vi "Simple Polar Plot.vi"() -> ()   [LabVIEW 2017]
doc: "Uses the Polar Plot with Point Options VI to draw a polar plot in a picture indicator."
panel:
  in  "Plot Color":u32(colorbox)=16715776
  in  "Grid Color":u32(colorbox)
  in  "Visible Section":u16(ring)=8
  in  "Stop":bool
  out "2D Picture":picture
  # "Overview: Demonstrates how to display and customize a polar plot using the Polar Plot with Point Options VI.\nInstructions:\n1. Run the VI.\n2. Change the Cosmetic Options to modify the visible area and appearance of the plot.\n3. Click Stop to stop the VI."
  # "Cosmetic Options"
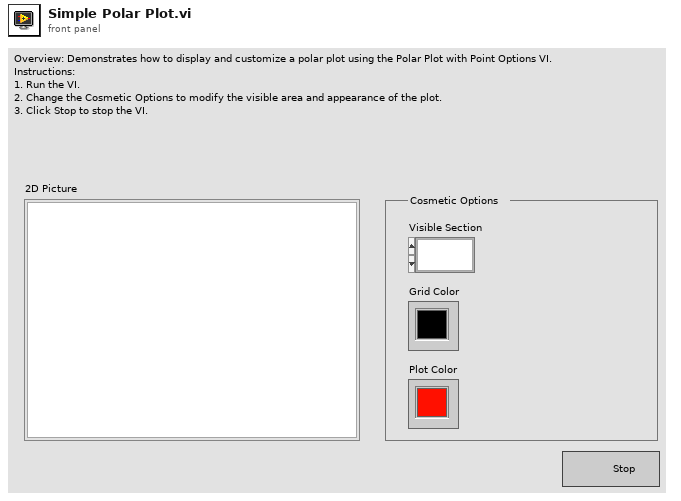
[diagram p1: front panel]
types:
  T1 = cluster{"maximum":dbl, "minimum":dbl, "clip to min":bool, "log?(F)":bool, "grid color":u32, "plot color":u32, "format and precision":cluster{"format":enum8{"Decimal", "Scientific", "Engineering", "Binary", "Octal", "Hex"}, "precision":u8}, "visible section":u16}
  T2 = typedef "LVBoundsTypeDef.ctl" = cluster{"Width":u32, "Height":u32}
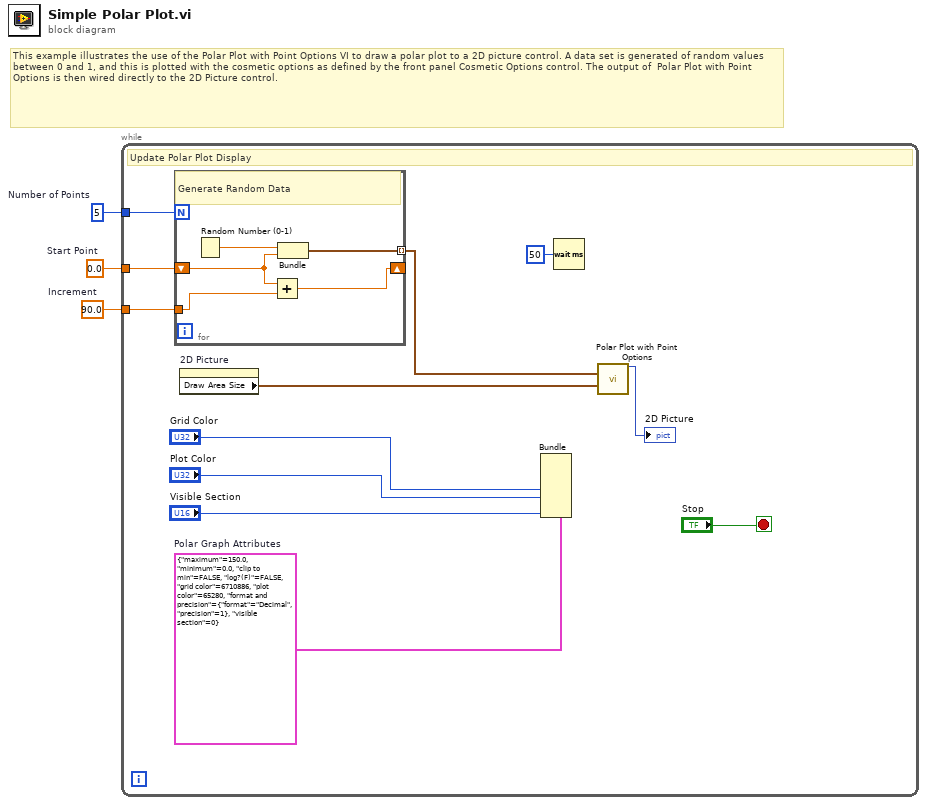
[diagram p0: block diagram]
diagram:
  w1 = 90.0  # Increment
  w2 = 0.0  # Start Point
  w3 = 5  # Number of Points
  # "This example illustrates the use of the Polar Plot with Point Options VI to draw a polar plot to a 2D picture control. A data set is generated of random values between 0 and 1, and this is plotted with the cosmetic options as defined by the front panel Cosmetic Options control. The output of  Polar Plot with Point Options is then wired directly to the 2D Picture control."
  n1 = while {
    tunnel: w3 -> [w15]
    tunnel: w2 -> [w14]
    tunnel: w1 -> [w11]
    stop <- "Stop" stop-if-true
    w12 = T1 {"maximum"=150.0, "minimum"=0.0, "clip to min"=FALSE, "log?(F)"=FALSE, "grid color"=6710886, "plot color"=65280, "format and precision"={"format"=enum."Decimal", "precision"=1}, "visible section"=0}  # Polar Graph Attributes
    # "Update Polar Plot Display"
    n2 = for {
      N: w15 -> [_]
      tunnel: [w20] -> w9 mode=indexing
      shift-right: [w19] -> _
      shift-left: w14 -> [w18]
      tunnel: w11 -> [w17]
      # "Generate Random Data"
      n3 = Random Number (0-1)() -> (number: 0 to 1=w16:dbl)
      n4 = Add(x=w18, y=w17) -> (x+y=w19:dbl)
      n5 = Bundle(w16, "Start Point"=w18) -> (w20:cluster{dbl, "Start Point":dbl})  [unwired: 1 in]
    }
    n6 = property on="2D Picture" class="Pict"() -> ("Draw Area Size"=w8:T2)  [unwired: 2 in, 2 out]
    n7 = Bundle(cluster=w12, "grid color"="Grid Color", "plot color"="Plot Color", "visible section"="Visible Section") -> ()  [unwired: 5 in, 1 out]
    n8 = Wait (ms)(milliseconds to wait=u32 50) -> ()  [unwired: 1 out]
    n9 = call <vilib>:"Polar Plot with Point Options.vi"("data array [mag, phase (deg)]"=w9, "dimensions (w,h)"=w8) -> ("new picture"=→"2D Picture":picture)  [unwired: 13 in]
  }
